vi "Timer Start.vi"(8 "error in (no error)":errorcluster, 11 "Timer reference":refnum<data-value>) -> (0 "error out":errorcluster, 3 "Timer reference  out":refnum<data-value>)   [LabVIEW 2009]
doc: "This VI is part of a Timer class that is implemented with the DVR. It starts the Timer. The Timer can be stopped and restared an infinite number of times. It's funtionality resembles a stopwatch\n\nAAL 9/09"
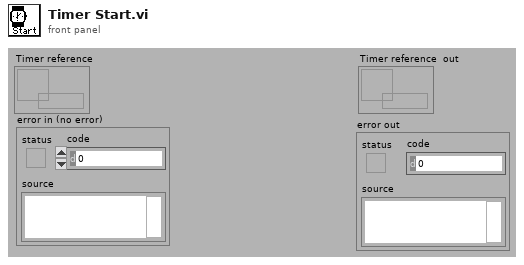
[diagram p1: front panel]
types:
  T1 = cluster{"Start Time":i32, "Elapsed Time":i32, "Running?":bool}
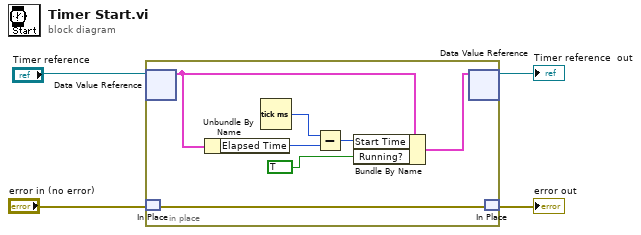
[diagram p0: block diagram]
diagram:
  n1 = in-place {
    n2 = in-place-dvr #1("Timer reference") -> (w7:T1)  [unwired: 1 out]
    n3 = in-place-match #2("error in (no error)") -> (w10:errorcluster)
    n4 = Unbundle By Name(w7) -> ("Elapsed Time"=w8:i32)
    n5 = Tick Count (ms)() -> (millisecond timer value=w9:u32)
    n6 = Subtract(x=w9, y=w8) -> (x-y=w6:u32)
    n7 = Bundle By Name(cluster=w7, "Start Time"=w6, "Running?"=TRUE) -> (w11:T1)
    n8 = in-place-dvr #1(w11) -> (→"Timer reference  out":refnum<data-value>)  [unwired: 1 out]
    n9 = in-place-match #2(w10) -> (→"error out":errorcluster)
  }
